vi "Measure Single Point With Compliance.vi"(8 "error in":errorcluster, 11 "niDMM in":refnum<class "niDMM.lvclass">) -> (0 "error out":errorcluster, 1 "Out_Of_Range":bool, 2 "Measured_Value":dbl, 3 "niDMM out":refnum<class "niDMM.lvclass">)   [LabVIEW 2020, in "niDMM.lvclass"]
uses:
  niDMM.lvclass
  niDMM.lvclass/niDMM.ctl
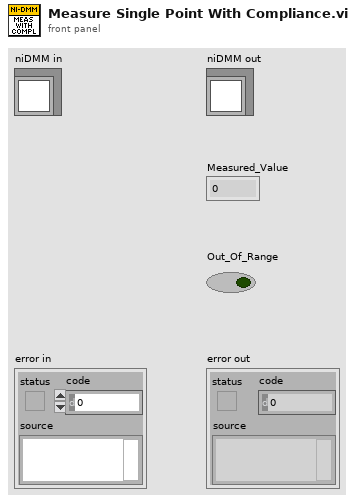
[diagram p1: front panel]
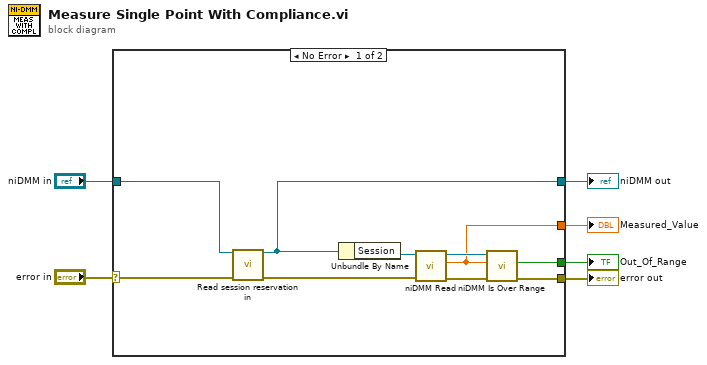
[diagram p0: block diagram]
diagram:
  n1 = case shown="No Error" "error in" {
    selector: "error in" -> [w13 w18]
    tunnel: [w12 w18] -> w5
    tunnel: "niDMM in" -> [w11 w17]
    tunnel: [w10 w17] -> w3
    tunnel: [w8 _] -> w2
    tunnel: [w7 _] -> w1
    frame No Error {
      n2 = call-dynamic "Read session reservation in.vi"("AbstractDMM in"=w11, "error in (no error)"=w13) -> ("AbstractDMM out"=w10:refnum<class "niDMM.lvclass">, "error out"=w9:errorcluster)  [unwired: 11 in, 1 out]
      n3 = Unbundle By Name(w10) -> ("Session"=w16:refnum<k15>)
      n4 = call <instrlib>:"niDMM Read.vi"("error in (no error)"=w9, "instrument handle"=w16) -> ("error out"=w14:errorcluster, "Measurement"=w7:dbl, "instrument handle out"=w15:refnum<k15>)  [unwired: 7 in]
      n5 = call <instrlib>:"niDMM Is Over Range.vi"("error in (no error)"=w14, "Measurement"=w7, "instrument handle"=w15) -> ("error out"=w12:errorcluster, "Over Range?"=w8:bool)  [unwired: 6 in, 1 out]
    }
    frame Error {
    }
  }
  "error out" <- w5
  "niDMM out" <- w3
  "Measured_Value" <- w1
  "Out_Of_Range" <- w2
